vi "LaunchStatus.vi"(8 "error in (no error)":errorcluster, 11 "Show Status?":bool) -> (0 "error out":errorcluster)   [LabVIEW 2018]
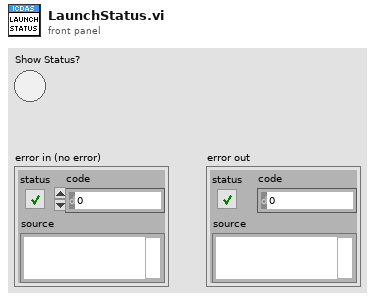
[diagram p1: front panel]
types:
  T1 = enum32{"Bad", "Idle", "Run top level", "Running"}
  T2 = enum32{"Invalid", "Standard", "Closed", "Hidden", "Minimized", "Maximized"}
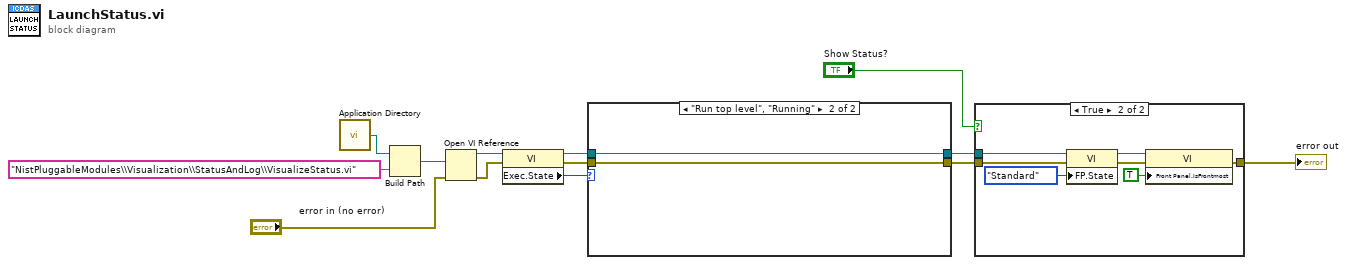
[diagram p0: block diagram]
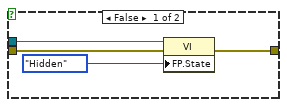
[diagram p2: hidden frame]
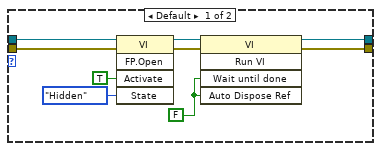
[diagram p3: hidden frame]
diagram:
  n1 = call <vilib>:"Application Directory.vi"() -> ("Application Directory"=w12:path)
  n2 = Build Path(base path=w12, name or relative path="NistPluggableModules\\Visualization\\StatusAndLog\\VisualizeStatus.vi") -> (appended path=w11:path)
  n3 = Open VI Reference(vi path=w11, error in (no error)="error in (no error)") -> (vi reference=w10:refnum<vi>, error out=w8:errorcluster)  [unwired: 4 in]
  n4 = property class="VI"(reference=w10, error in=w8) -> (reference out=w9:refnum<vi>, error out=w7:errorcluster, "Exec.State"=w6:T1)
  n5 = case shown="\"Run top level\", \"Running\"" w6 {
    tunnel: w9 -> [w17 w24]
    tunnel: w7 -> [w16 w23]
    tunnel: [w15 w23] -> w3
    tunnel: [w14 w24] -> w4
    frame Default {
      w20 = FALSE ("Wait Until Done")
      n6 = invoke class="VI" method="FP.Open"(reference=w17, error in=w16, "Activate"=TRUE ("Activate?"), "State"=T2."Hidden") -> (reference out=w19:refnum<vi>, error out=w18:errorcluster)  [unwired: 1 in, 3 out]
      n7 = invoke class="VI" method="Run VI"(reference=w19, error in=w18, "Wait until done"=w20, "Auto Dispose Ref"=w20) -> (reference out=w14:refnum<vi>, error out=w15:errorcluster)  [unwired: 1 in, 3 out]
    }
    frame "Run top level", "Running" {
    }
  }
  n8 = case shown="True" "Show Status?" {
    tunnel: w4 -> [w28 w31]
    tunnel: w3 -> [w27 w34]
    tunnel: [w25 w33] -> w2
    frame False {
      n9 = property class="VI"(reference=w28, error in=w27, "FP.State"=T2."Hidden" ("Front Panel Window:State")) -> (error out=w25:errorcluster)  [unwired: 1 out]
    }
    frame True {
      n10 = property class="VI"(reference=w31, error in=w34, "FP.State"=T2."Standard" ("Front Panel Window:State")) -> (reference out=w30:refnum<vi>, error out=w32:errorcluster)
      n11 = property class="VI"(reference=w30, error in=w32, "Front Panel.IsFrontmost"=TRUE ("Front Panel Window:Is Frontmost")) -> (error out=w33:errorcluster)  [unwired: 1 out]
    }
  }
  "error out" <- w2
